vi "PythonError.vi"(6 "reply":string, 8 "error in (no error)":errorcluster, 10 "function name":string) -> (0 "error out":errorcluster)   [LabVIEW 2022 SP3]
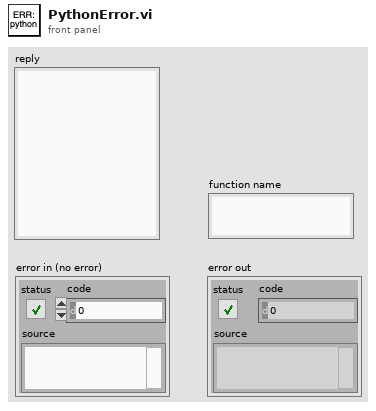
[diagram p1: front panel]
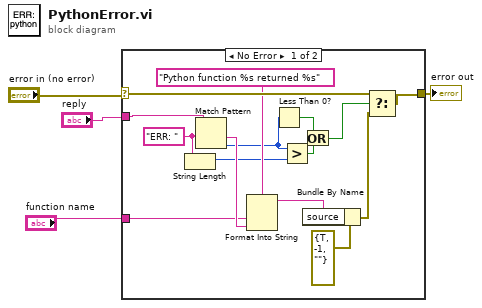
[diagram p0: block diagram]
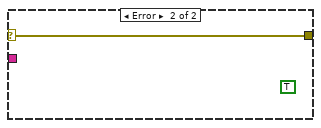
[diagram p2: hidden frame]
diagram:
  n1 = case shown="No Error" "error in (no error)" {
    selector: "error in (no error)" -> [w18 w20]
    tunnel: "reply" -> [w16 _]
    tunnel: [w19 w20] -> w4
    tunnel: "function name" -> [w12 _]
    frame No Error {
      w10 = "ERR: " ("function name")
      n2 = String Length(string=w10) -> (length=w8:i32)
      n3 = Match Pattern(string=w16, regular expression=w10) -> (after substring=w13:string, offset past match=w9:i32)  [unwired: 1 in, 2 out]
      n4 = Format Into String(format string="Python function %s returned %s", w12, w13) -> (resulting string=w11:string)  [unwired: 2 in, 1 out]
      n5 = Less Than 0?(x=w9) -> (x < 0?=w7:bool)
      n6 = Greater?(x=w9, y=w8) -> (0:w6:bool)
      n7 = Or(x=w7, y=w6) -> (x .or. y?=w5:bool)
      n8 = Bundle By Name(cluster=errorcluster {"status"=TRUE, "code"=-1, "source"=""} ("f"), "source"=w11) -> (w15:errorcluster)
      n9 = Select(t=w18, s=w5, f=w15) -> (s? t:f=w19:errorcluster)
    }
    frame Error {
      (unwired) TRUE
    }
  }
  "error out" <- w4
